vi "Resistance_to_Temp_Conversion(SubVI).vi"(11 "Scalar":dbl) -> (3 "Result":dbl)   [LabVIEW 2012]
uses:
  <vilib>/express/express arith-compare/Formula/XNode/ExpressFormulaBlockNode.xnode
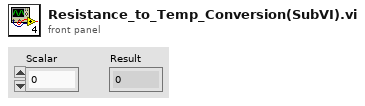
[diagram p1: front panel]
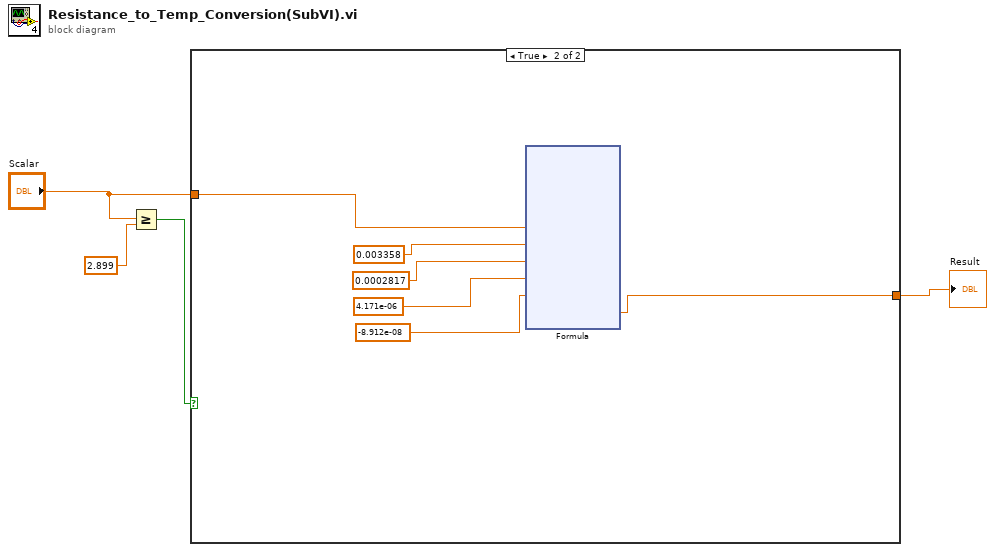
[diagram p0: block diagram]
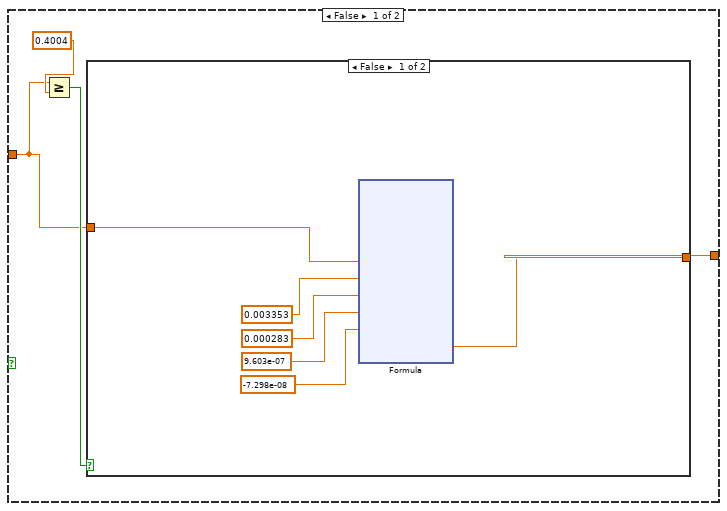
[diagram p2: hidden frame]
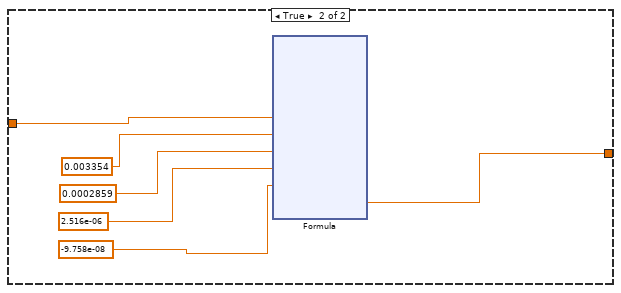
[diagram p3: hidden frame]
diagram:
  n1 = Greater Or Equal?(x="Scalar", y=2.899) -> (x >= y?=w1:bool)
  n2 = case shown="True" w1 {
    tunnel: "Scalar" -> [w5 w58]
    tunnel: [w8 w53] -> w2
    frame False {
      n3 = Greater Or Equal?(x=w5, y=0.4004) -> (x >= y?=w7:bool)
      n4 = case shown="False" w7 {
        tunnel: w5 -> [w14 w36]
        tunnel: [w13 w31] -> w8
        frame False {
          n5 = xnode "Formula"("Ratio"=w14, "a"=0.003353, "b"=0.000283, "c"=9.603e-07, "d"=-7.298e-08) -> ("Result"=w13:dbl)  [unwired: 1 in, 1 out]
        }
        frame True {
          n6 = xnode "Formula"("Ratio"=w36, "a"=0.003354, "b"=0.0002859, "c"=2.516e-06, "d"=-9.758e-08) -> ("Result"=w31:dbl)  [unwired: 1 in, 1 out]
        }
      }
    }
    frame True {
      n7 = xnode "Formula"("Ratio"=w58, "a"=0.003358, "b"=0.0002817, "c"=4.171e-06, "d"=-8.912e-08) -> ("Result"=w53:dbl)  [unwired: 1 in, 1 out]
    }
  }
  "Result" <- w2
